vi "SVT Belts.vi"(0 "pulley1 pitch diameter":dbl=1.0, 1 "pulley1 nominal speed [RPM]":dbl=1200.0, 2 "desired units":u16(ring) items=["Hz", "Order"], 5 "pulley2 pitch diameter":dbl=2.0, 7 "center distance":dbl=10.0, 11 "error in (no error)":errorcluster, 12 "teeth parameters":cluster{"type":u16, "number of teeth":u32}={"type"=0, "number of teeth"=37} {"type" items=["Belt Teeth", "Pulley1 Teeth", "Pulley2 Teeth"]}) -> (3 "pulley2 nominal speed [RPM]":dbl=600.0, 4 "pulley1 misalign/eccen frequency":dbl=20.0, 6 "pulley2 misalign/eccen frequency":dbl=10.0, 8 "belt frequency":dbl=2.539956531342396, 10 "timing belt frequency":dbl=93.97839165966865, 14 "belt length":dbl=24.73737337488548, 15 "error out":errorcluster)   [LabVIEW 2017, in "SoundVib_MachineCharacteristic.lvlib"]
doc: "Calculates characteristic frequencies or orders of belts."
uses:
  <vilib>/addons/Sound and Vibration/svt_Machine Characteristic/SoundVib_MachineCharacteristic.lvlib
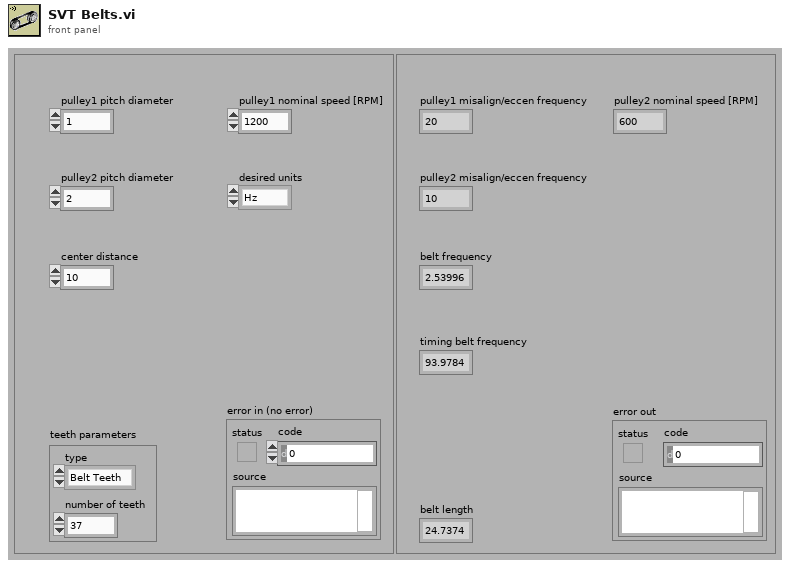
[diagram p1: front panel]
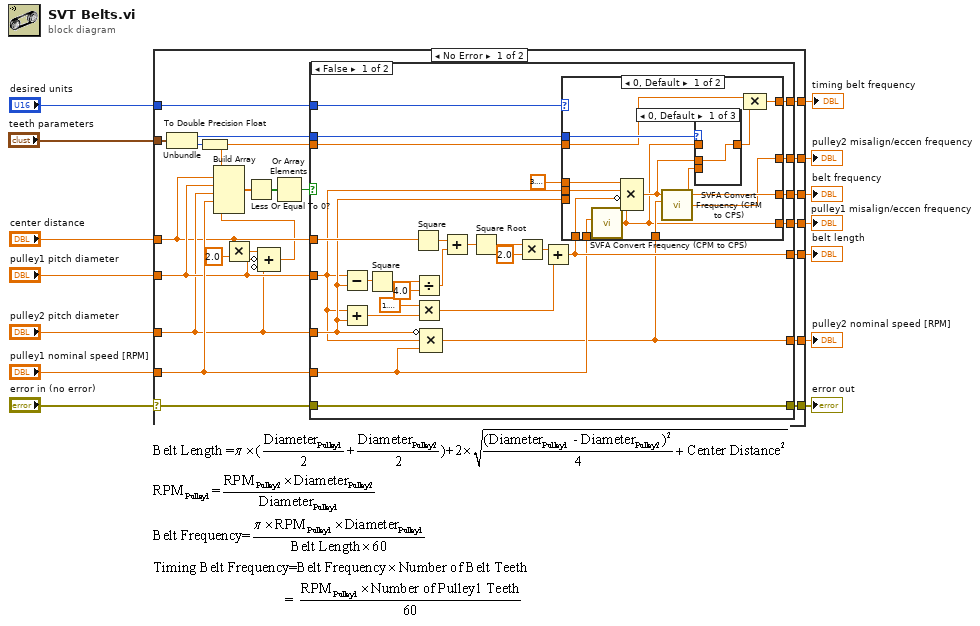
[diagram p0: block diagram]
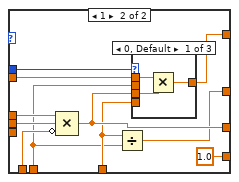
[diagram p4: hidden frame]
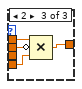
[diagram p6: hidden frame]
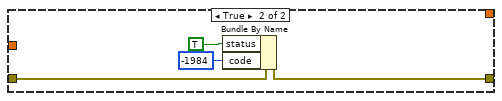
[diagram p7: hidden frame]
diagram:
  n1 = case shown="No Error" "error in (no error)" {
    selector: "error in (no error)" -> [w35 w103]
    tunnel: [w34 w103] -> w13
    tunnel: "pulley1 pitch diameter" -> [w20 _]
    tunnel: "pulley2 pitch diameter" -> [w19 _]
    tunnel: "center distance" -> [w18 _]
    tunnel: [w37 _] -> w9
    tunnel: "pulley1 nominal speed [RPM]" -> [w26 _]
    tunnel: [w36 _] -> w7
    tunnel: "desired units" -> [w33 _]
    tunnel: [w32 _] -> w5
    tunnel: "teeth parameters" -> [w31 _]
    tunnel: [w29 _] -> w3
    tunnel: [w22 _] -> w2
    tunnel: [w21 _] -> w1
    frame No Error {
      n2 = Unbundle(w31) -> ("type"=w30:u16, "number of teeth"=w28:u32)
      n3 = To Double Precision Float(number=w28) -> (double precision float=w27:dbl)
      n4 = Multiply(x=w18, y=2.0) -> (x*y=w17:dbl)
      n5 = Compound Arithmetic op=ADD(w17, invert w20, invert w19) -> (w15:dbl)
      n6 = Build Array(w27, w18, w20, w19, w26, w15) -> (w25:dbl[])
      n7 = Less Or Equal To 0?(x=w25) -> (x <= 0?=w24:bool[])
      n8 = Or Array Elements(Boolean array=w24) -> (logical OR=w23:bool)
      n9 = case shown="False" w23 {
        tunnel: [w49 _] -> w37
        tunnel: [w41 _] -> w36
        tunnel: w18 -> [w52 _]
        tunnel: w20 -> [w44 _]
        tunnel: w19 -> [w45 _]
        tunnel: w26 -> [w43 _]
        tunnel: w35 -> [w51 w102]
        tunnel: [w51 w101] -> w34
        tunnel: w33 -> [w50 _]
        tunnel: [w48 _] -> w32
        tunnel: w30 -> [w46 _]
        tunnel: w27 -> [w40 _]
        tunnel: [w42 _] -> w29
        tunnel: [w39 _] -> w22
        tunnel: [w38 _] -> w21
        frame False {
          n10 = Subtract(x=w44, y=w45) -> (x-y=w62:dbl)
          n11 = Add(x=w44, y=w45) -> (x+y=w64:dbl)
          n12 = Square(x=w62) -> (x^2=w61:dbl)
          n13 = Square(x=w52) -> (x^2=w59:dbl)
          n14 = Divide(x=w61, y=4.0) -> (x/y=w58:dbl)
          n15 = Multiply(x=1.5707963267948966, y=w64) -> (x*y=w53:dbl)
          n16 = Compound Arithmetic op=MULTIPLY(invert w45, w44, w43) -> (w41:dbl)
          n17 = Add(x=w59, y=w58) -> (x+y=w57:dbl)
          n18 = Square Root(x=w57) -> (sqrt(x)=w56:dbl)
          n19 = Multiply(x=w56, y=2.0) -> (x*y=w54:dbl)
          n20 = Add(x=w54, y=w53) -> (x+y=w49:dbl)
          n21 = case shown="0, Default" w50 {
            tunnel: w44 -> [w76 w88]
            tunnel: w43 -> [w69 w81]
            tunnel: w49 -> [w75 w90]
            tunnel: [w68 w84] -> w48
            tunnel: 3.141592653589793 -> [w74 w89]
            tunnel: w46 -> [w73 w87]
            tunnel: w45 -> [_ _]
            tunnel: w40 -> [w72 w86]
            tunnel: [w70 w85] -> w42
            tunnel: w41 -> [w67 w82]
            tunnel: [w65 1.0] -> w39
            tunnel: [w66 w80] -> w38
            frame 0, Default {
              n22 = call <vilib>:"SVFA Convert Frequency (CPM to CPS).vi"("nominal speed [RPM]"=w69) -> ("frequency [Hz]"=w65:dbl)  [unwired: 5 in]
              n23 = Compound Arithmetic op=MULTIPLY(w74, w76, invert w75, w65) -> (w68:dbl)
              n24 = call <vilib>:"SVFA Convert Frequency (CPM to CPS).vi"("nominal speed [RPM]"=w67) -> ("frequency [Hz]"=w66:dbl)  [unwired: 5 in]
              n25 = case shown="0, Default" w73 {
                tunnel: w68 -> [w77 _ _]
                tunnel: [w77 w78 w79] -> w71
                tunnel: w66 -> [_ _ w79]
                tunnel: w65 -> [_ w78 _]
                frame 0, Default {
                }
                frame 1 {
                }
                frame 2 {
                }
              }
              n26 = Compound Arithmetic op=MULTIPLY(w72, w71) -> (w70:dbl)
            }
            frame 1 {
              n27 = Compound Arithmetic op=MULTIPLY(w89, w88, invert w90) -> (w84:dbl)
              n28 = Divide(x=w82, y=w81) -> (x/y=w80:dbl)
              n29 = case shown="0, Default" w87 {
                tunnel: w86 -> [w93 w94 w98]
                tunnel: w84 -> [w92 _ _]
                tunnel: [w91 w94 w95] -> w85
                tunnel: w81 -> [_ _ w96]
                tunnel: w82 -> [_ _ w97]
                frame 0, Default {
                  n30 = Multiply(x=w93, y=w92) -> (x*y=w91:dbl)
                }
                frame 1 {
                }
                frame 2 {
                  n31 = Compound Arithmetic op=MULTIPLY(w98, invert w96, w97) -> (w95:dbl)
                }
              }
            }
          }
        }
        frame True {
          n32 = Bundle By Name(cluster=w102, "status"=TRUE, "code"=-1984) -> (w101:errorcluster)
        }
      }
    }
    frame Error {
    }
  }
  "belt frequency" <- w5
  "belt length" <- w9
  "pulley2 nominal speed [RPM]" <- w7
  "timing belt frequency" <- w3
  "error out" <- w13
  "pulley1 misalign/eccen frequency" <- w2
  "pulley2 misalign/eccen frequency" <- w1
